vi "FTW-Publisher-Listener-Start.vi"(0 "FTW Publisher in":refnum<class "FTW-Publisher.lvclass">, 5 "FTW Endpoint":refnum<class "FTW-Endpoint.lvclass">, 7 "Send Timeout":i32, 9 "Send Buffer Depth":i32, 11 "error in (no error)":errorcluster) -> (4 "FTW Publisher out":refnum<class "FTW-Publisher.lvclass">, 15 "error out":errorcluster)   [LabVIEW 2013, in "FTW-Publisher.lvclass"]
uses:
  FTW-Publisher.lvclass
  Endpoint/FTW-Endpoint.lvclass
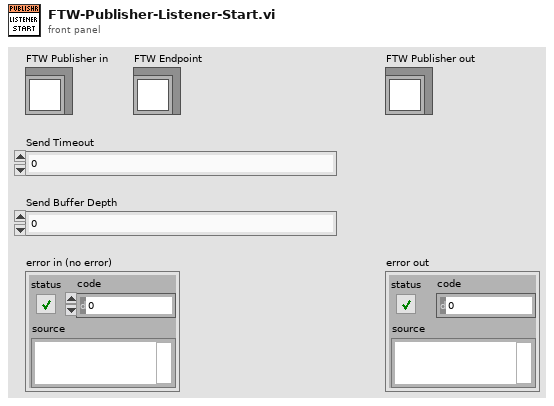
[diagram p1: front panel]
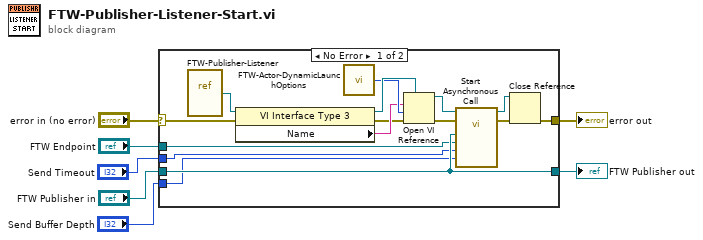
[diagram p0: block diagram]
diagram:
  n1 = case shown="No Error" "error in (no error)" {
    selector: "error in (no error)" -> [w21 w23]
    tunnel: [w22 w24] -> w7
    tunnel: "FTW Publisher in" -> [w22 w24]
    tunnel: "Send Buffer Depth" -> [w20 _]
    tunnel: "Send Timeout" -> [w19 _]
    tunnel: [w17 w23] -> w2
    tunnel: "FTW Endpoint" -> [w8 _]
    frame No Error {
      n2 = vi-ref "FTW-Publisher-Listener.vi"() -> (w9:refnum<vi>)
      n3 = property class="VI Interface Type 3"(reference=w9, error in=w21) -> (reference out=w13:refnum<vi>, error out=w10:errorcluster, "Name"=w11:string)
      n4 = call "FTW-Actor-DynamicLaunchOptions.vi"() -> ("Open VI Ref Options"=w12:i32)
      n5 = Open VI Reference(type specifier VI Refnum (for type only)=w13, vi path=w11, options=w12, error in (no error)=w10) -> (vi reference=w15:refnum<vi>, error out=w18:errorcluster)  [unwired: 2 in]
      n6 = call-by-ref "Start Asynchronous Call"(reference=w15, error in=w18, "keep most recent"=w20, "Timeout"=w19, "FTW Endpoint"=w8, "FTW Publisher"=w22) -> (reference out=w16:refnum<vi>, error out=w14:errorcluster)  [unwired: 1 in]
      n7 = Close Reference(reference=w16, error in (no error)=w14) -> (error out=w17:errorcluster)
    }
    frame Error {
    }
  }
  "FTW Publisher out" <- w7
  "error out" <- w2
